vi "Environment Step Type - Set Environment.vi"(9 "Value":dbl, 10 "Setting":T1, 11 "Sequence Context In":refnum<k7>) -> (0 "error out":errorcluster, 1 "Commited Value":dbl)   [LabVIEW 2013]
uses:
  <instrlib>/Driver Simulation/Fixture/EnvironmentSettings.ctl
  <instrlib>/Driver Simulation/Fixture.lvlib
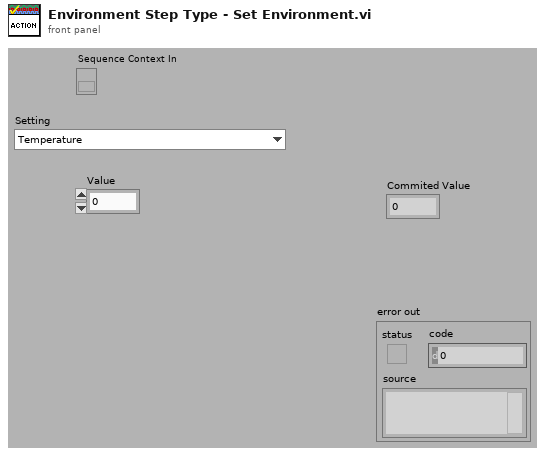
[diagram p1: front panel]
types:
  T1 = typedef "Driver Simulation.lvlib/Fixture.lvlib/EnvironmentSettings.ctl" = enum16{"Temperature", "Light Intensity"}
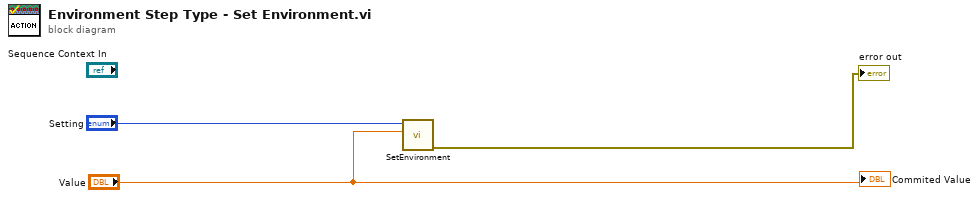
[diagram p0: block diagram]
diagram:
  n1 = call <instrlib>:"SetEnvironment.vi"("Value"="Value", "Setting"="Setting") -> ("error out"=→"error out":errorcluster)  [unwired: 9 in]
  "Commited Value" <- "Value"
